vi "trigger_echo.vi"() -> ()   [LabVIEW 2019]
uses:
  <vilib>/rvi/Emulation/niFpgaGetClockAttributes.vi
  <vilib>/rvi/Emulation/niFpgaSctlEmulationGetInTimedLoop.vi
  <vilib>/rvi/Emulation/niFpgaEmulationReportErrorSimple.vi
  <vilib>/rvi/eio/common/nirviEmuTemplateMethod_errors.vi
  <vilib>/rvi/Emulation/niFpgaCriticalErrorInLSC.vi
  <vilib>/eio/EIONode/EIONode.xnode
panel:
  out "Meter":i16(knob) scale=0.0..200.0
  in  "Echo stop":bool
  out "Jarak":i32
  in  "Trigger stop button":bool
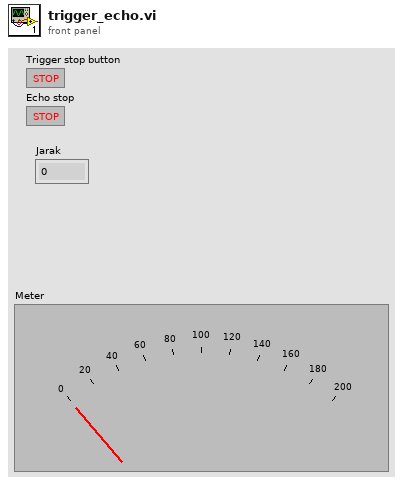
[diagram p1: front panel]
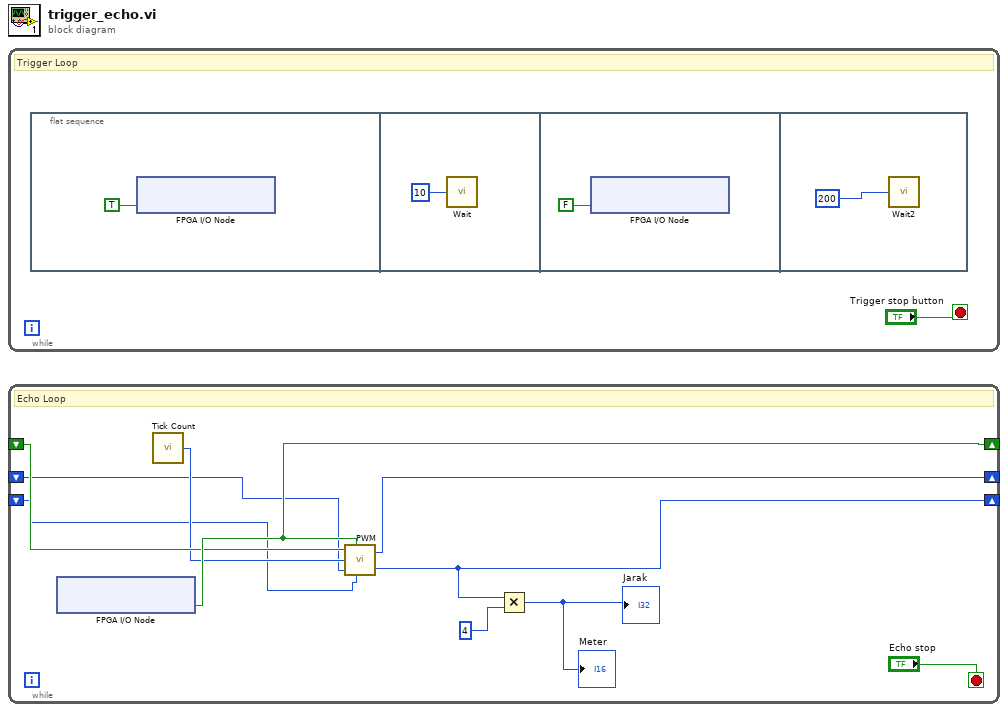
[diagram p0: block diagram]
diagram:
  n1 = while {
    stop <- "Trigger stop button" stop-if-true
    # "Trigger Loop"
    n2 = flat-sequence {
      frame #0 {
        n3 = xnode "FPGA I/O Node"("ConnectorC/DIO5"=TRUE) -> ()  [unwired: 1 in, 1 out]
      }
      frame #1 {
        n4 = call "Wait"("Count(uSec)"=u32 10) -> ()  [unwired: 1 out]
      }
      frame #2 {
        n5 = xnode "FPGA I/O Node"("ConnectorC/DIO5"=FALSE) -> ()  [unwired: 1 in, 1 out]
      }
      frame #3 {
        n6 = call "Wait2"("Count(uSec)"=u32 200) -> ()  [unwired: 1 out]
      }
    }
  }
  n7 = while {
    shift-right: [w15] -> _
    shift-left: _ -> [w14]
    shift-right: [w10] -> _
    shift-left: _ -> [w12]
    shift-right: [w9] -> _
    shift-left: _ -> [w11]
    stop <- "Echo stop" stop-if-true
    # "Echo Loop"
    n8 = xnode "FPGA I/O Node"() -> ("ConnectorC/DIO6"=w15:bool)  [unwired: 1 in, 1 out]
    n9 = call "Tick Count"() -> ("Tick Count(mSec)"=w13:u32)
    n10 = call "PWM.vi"("Echo Sebelum"=w14, "Echo Saat Ini"=w15, "Tick Saat Ini"=w13, "PWM Input Saat Ini"=w12, "PWM Input Sebelum"=w11) -> ("PWM Output Saat Ini"=w10:i32, "PWM Output"=w9:i32)
    n11 = Multiply(x=w9, y=4) -> (x*y=→"Jarak" →"Meter":i32)
  }
